vi "sub_check_and_autocreate_event.vi"(8 "error in (no error)":errorcluster, 9 "new Event Label":string, 10 "Event Key to Create or Update":string, 11 "daq.io type in in":T1={"daq.io ref"=refnum, "daq.io API Base"="", "Device Type Key"="", "Device Key"="", "Account ID"="", "online"=TRUE}) -> (0 "error out":errorcluster, 1 "found at index":i32, 3 "daq.io type out":T1={"daq.io ref"=refnum, "daq.io API Base"="", "Device Type Key"="", "Device Key"="", "Account ID"="", "online"=TRUE})   [LabVIEW 2013, in "daqio minimal.lvlib"]
doc: "This VI autocreates a new Event Type if required."
uses:
  daqio minimal.lvlib
  _typedefs/daqio-Type.ctl
  <vilib>/httpClient/ClientHandle.ctl
  _typedefs/FGV_commands.ctl
  <vilib>/httpClient/LabVIEWHTTPClient.lvlib
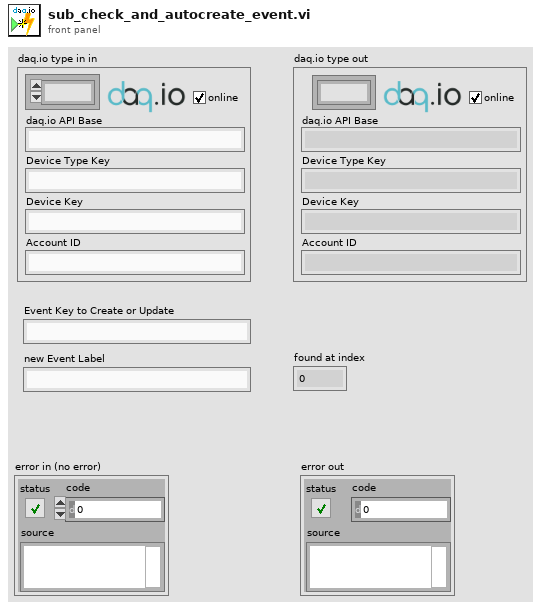
[diagram p1: front panel]
types:
  T1 = typedef "daqio minimal.lvlib/daqio-Type.ctl" = cluster{"daq.io ref":T2, "daq.io API Base":string, "Device Type Key":string, "Device Key":string, "Account ID":string, "online":bool}
  T2 = typedef "LabVIEWHTTPClient.lvlib/ClientHandle.ctl" = refnum<k1>
  T3 = typedef "daqio minimal.lvlib/FGV_commands.ctl" = enum16{"Init / update", "Edit Item", "Find or Add Item", "Remove Item", "Delete All"}
  T4 = typedef "daqio minimal.lvlib/daqio-Device-Type-Info-return.ctl" = cluster{"channel_types":T5[], "devices":T6[], "label":string, "event_types":T7[], "key":string, "tag_types":T8[], "id":string, "permissions":cluster{"write":string[], "read":string[]}}
  T5 = typedef "daqio minimal.lvlib/daqio-Channel-Type-POST-return.ctl" = cluster{"device_type_id":string, "id":string, "key":string, "label":string, "data_type":string, "permissions":cluster{"write":string[], "read":string[]}}
  T6 = typedef "daqio minimal.lvlib/daqio-Device.ctl" = cluster{"permissions":cluster{"write":string[], "read":string[]}, "id":string, "label":string, "key":string, "device_type_id":string, "tags":cluster{"key":string, "value":string}[], "files":string[]}
  T7 = typedef "daqio minimal.lvlib/daqio-Event-Type.ctl" = cluster{"device_type_id":string, "permissions":cluster{"read":string[], "write":string[]}, "id":string, "key":string, "label":string}
  T8 = typedef "daqio minimal.lvlib/daqio-Tag-Type-POST-return.ctl" = cluster{"label":string, "id":string, "device_type_id":string, "permissions":cluster{"write":string[], "read":string[]}, "default":string, "key":string}
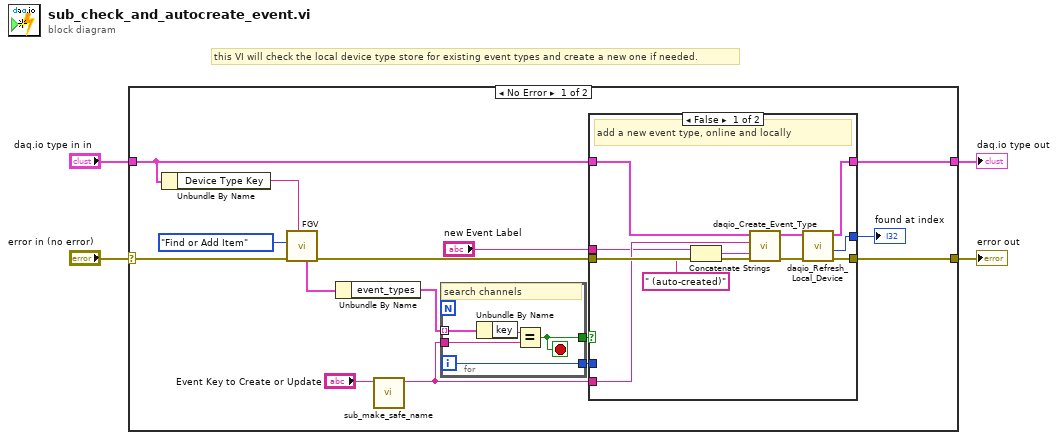
[diagram p0: block diagram]
diagram:
  # "this VI will check the local device type store for existing event types and create a new one if needed."
  n1 = case shown="No Error" "error in (no error)" {
    selector: "error in (no error)" -> [w10 w40]
    tunnel: [w12 w40] -> w4
    tunnel: [w11 w39] -> w3
    tunnel: "daq.io type in in" -> [w9 w39]
    frame No Error {
      n2 = Unbundle By Name(w9) -> ("Device Type Key"=w8:string)
      n3 = call "FGV.vi"("Dev Type Key"=w8, "error in (no error)"=w10, "Action"=FGV_commands."Find or Add Item") -> ("error out"=w17:errorcluster, "Dev Type out"=w18:T4)  [unwired: 4 in, 3 out]
      n4 = Unbundle By Name(w18) -> ("event_types"=w15:T7[])
      n5 = call "sub_make_safe_name.vi"("Input String"="Event Key to Create or Update") -> ("Safe Output String"=w19:string)  [unwired: 10 in]
      n6 = for {
        tunnel: w15 -> [w38] mode=indexing
        tunnel: w19 -> [w36]
        tunnel: [w35] -> w16
        tunnel: [w34] -> w6
        i -> [w34]
        stop <- w35 stop-if-true
        # "search channels"
        n7 = Unbundle By Name(w38) -> ("key"=w37:string)
        n8 = Equal?(x=w37, y=w36) -> (x = y?=w35:bool)
      }
      n9 = case shown="False" w16 {
        tunnel: w9 -> [w26 w33]
        tunnel: [w30 w33] -> w11
        tunnel: w19 -> [w27 _]
        tunnel: w17 -> [w28 w32]
        tunnel: [w29 w32] -> w12
        tunnel: [w23 w31] -> w7
        tunnel: w6 -> [_ w31]
        tunnel: "new Event Label" -> [w21 _]
        frame False {
          # "add a new event type, online and locally"
          n10 = Concatenate Strings(w21, " (auto-created)" ("string")) -> (w22:string)
          n11 = call "daqio_Create_Event_Type.vi"("error in (no error)"=w28, "new Event Label"=w22, "new Event Key"=w27, "daq.io type in"=w26) -> ("error out"=w24:errorcluster, "daq.io type out"=w25:T1)  [unwired: 5 in, 1 out]
          n12 = call "daqio_Refresh_Local_Device.vi"("error in (no error)"=w24, "daq.io type in"=w25) -> ("error out"=w29:errorcluster, "found at index"=w23:i32, "daq.io type out"=w30:T1)  [unwired: 5 in, 2 out]
        }
        frame True {
          # "don't add anything, it exists"
        }
      }
      "found at index" <- w7
    }
    frame Error {
    }
  }
  "error out" <- w4
  "daq.io type out" <- w3
